vi "未命名 1 (子VI).vi"() -> ()   [LabVIEW 2016, in "质控单元.lvlib"]
panel:
  in  "字符串":string
  out "子数组 2":u16[](array[numeric]) format="%x"
  out "子数组":u16[](array[numeric]) format="%x"
  out "数组 2":u16[](array[numeric]) format="%x"
  out "文本":string
  out "JSON字符串 2":string
  in  "JSON字符串":string
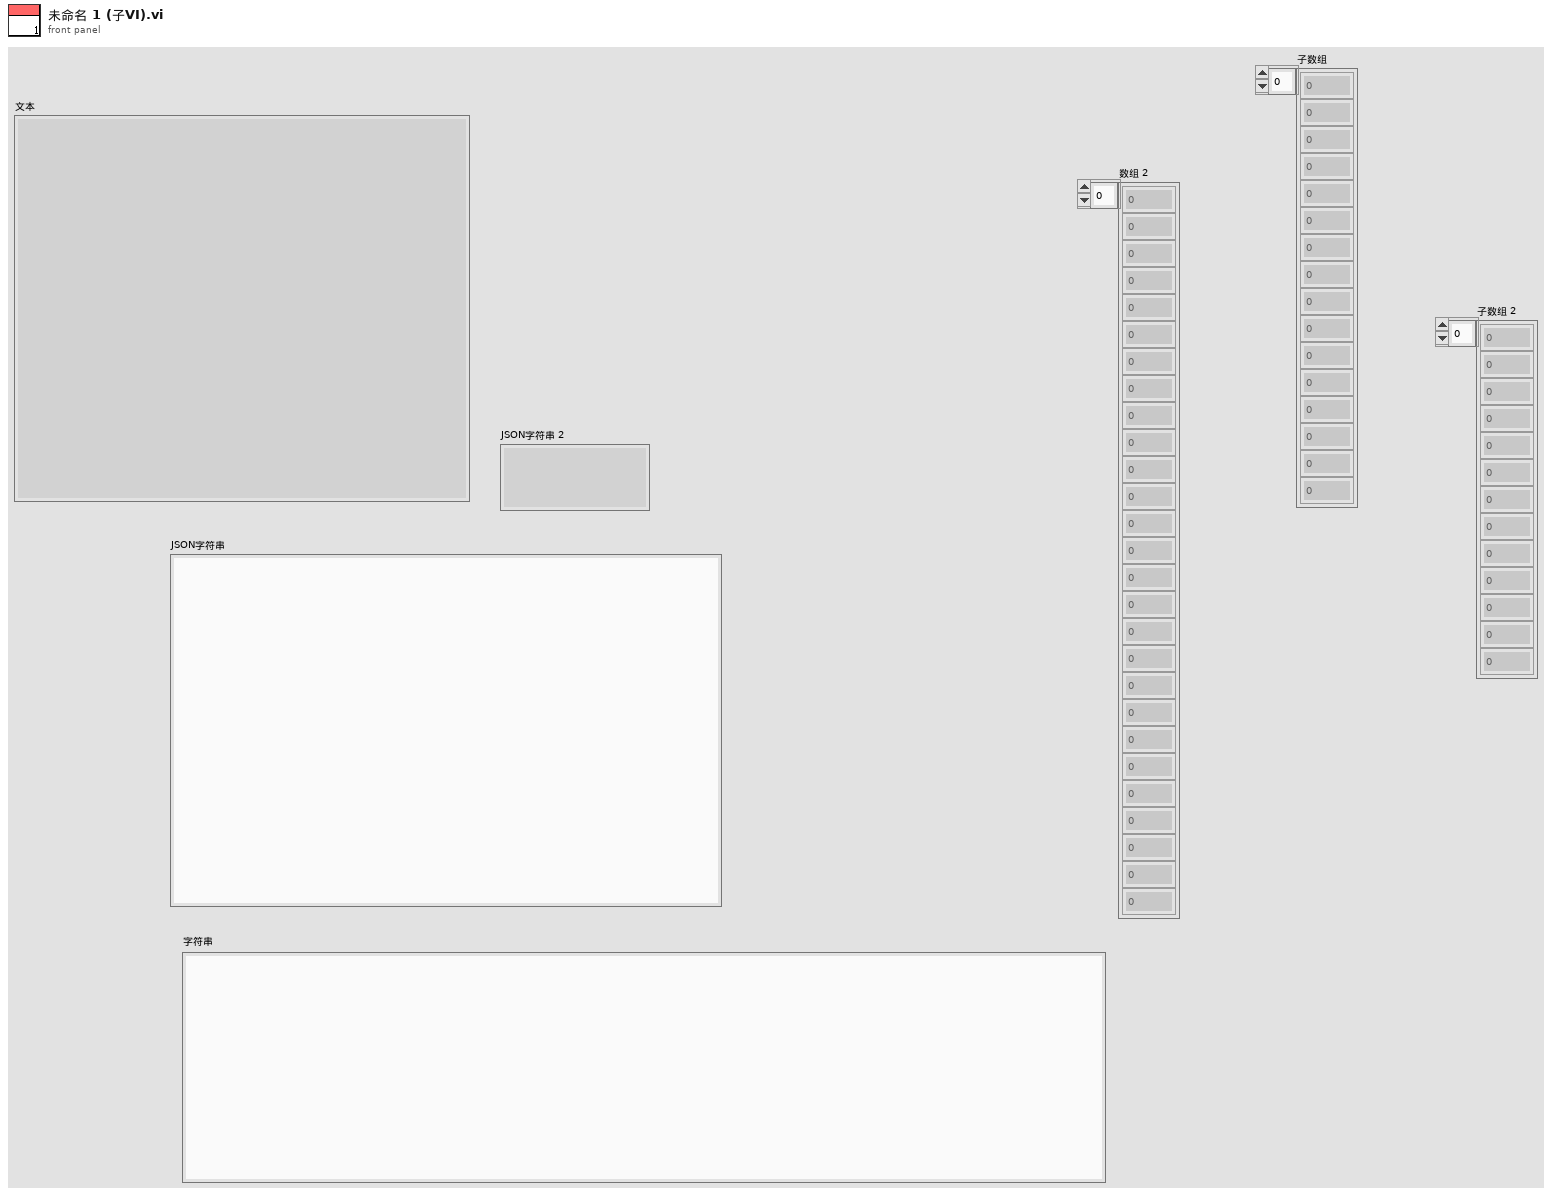
[diagram p1: front panel]
types:
  T1 = cluster{"flow1":cluster{"Type":u16, "Value":sgl}[], "flow2":cluster{"Type":u16, "Value":sgl}[], "flow3":cluster{"Type":u16, "Value":sgl}[]}
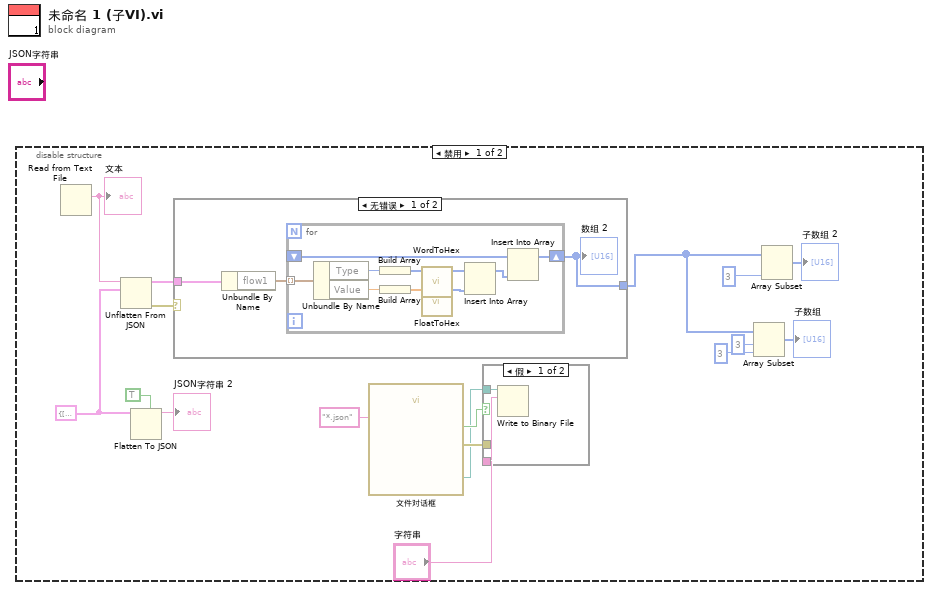
[diagram p0: block diagram]
diagram:
  n1 = disable-structure shown="禁用" {
    frame Disabled {
      w15 = T1 {"flow1"=[], "flow2"=[], "flow3"=[]}
      n2 = Read from Text File() -> (text=w14:string)  [unwired: 4 in, 3 out]
      "文本" <- w14
      n3 = Unflatten From JSON(JSON string=w14, type and defaults=w15) -> (value=w12:T1, error out=w13:errorcluster)  [unwired: 5 in]
      n4 = Flatten To JSON(enable LabVIEW extensions? (T)=TRUE ("启用LabVIEW扩展？(T)"), anything=w15) -> (JSON string=→"JSON字符串 2":string)  [unwired: 1 in, 1 out]
      n5 = case shown="无错误" w13 {
        tunnel: w12 -> [w22 _]
        tunnel: [w20 _] -> w8
        frame No Error {
          n6 = Unbundle By Name(w22) -> ("flow1"=w21:cluster{"Type":u16, "Value":sgl}[])
          n7 = for {
            tunnel: w21 -> [w32] mode=indexing
            shift-right: [w24] -> w20
            shift-left: _ -> [w23]
            n8 = Unbundle By Name(w32) -> ("Type"=w31:u16, "Value"=w29:sgl)
            n9 = Build Array(w31) -> (w30:u16[])
            n10 = Build Array(w29) -> (w28:sgl[])
            n11 = call "WordToHex.vi"("WORD"=w30) -> ("数组"=w27:u16[])  [unwired: 10 in]
            n12 = call "FloatToHex.vi"("浮点数"=w28) -> ("DCBA整形输出"=w26:u16[])  [unwired: 10 in]
            n13 = Insert Into Array(array=w27, new element=w26) -> (w25:u16[])  [unwired: 1 in]
            n14 = Insert Into Array(array=w23, new element=w25) -> (w24:u16[])  [unwired: 1 in]
          }
          "数组 2" <- w20
        }
        frame Error {
        }
      }
      n15 = call "文件对话框"("pattern (all files)"="*.json") -> ("selected path"=w2:path, "cancelled"=w4:bool, "error out"=w5:errorcluster)  [unwired: 11 in, 1 out]
      n16 = case shown="假" w4 {
        tunnel: w2 -> [w19 _]
        tunnel: "字符串" -> [w18 _]
        tunnel: w5 -> [_ _]
        frame False {
          n17 = Write to Binary File(file (use dialog)=w19, data=w18) -> ()  [unwired: 4 in, 3 out]
        }
        frame True {
        }
      }
      n18 = Array Subset(array=w8, index=3 ("索引"), length=3 ("长度")) -> (→"子数组":u16[])
      n19 = Array Subset(array=w8, length=3 ("长度")) -> (→"子数组 2":u16[])  [unwired: 1 in]
    }
    frame Enabled {
    }
  }
